vi "PWM Motor Control.vi"() -> ()   [LabVIEW 2010]
panel:
  out "Square":dynamicdata(graph)
  in  "Duty Cycle (%)":dbl=50.0
  in  "stop":bool
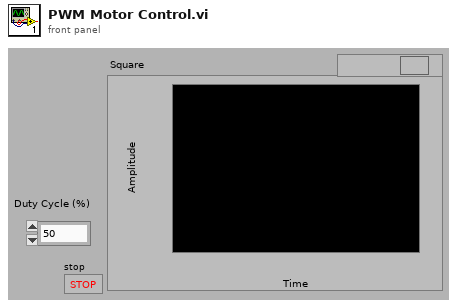
[diagram p1: front panel]
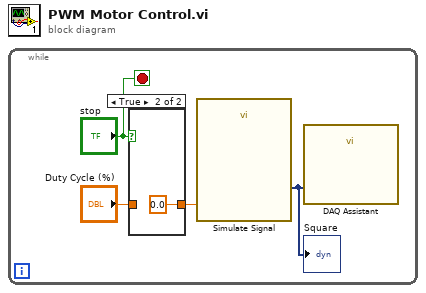
[diagram p0: block diagram]
diagram:
  n1 = while {
    stop <- "stop" stop-if-true
    n2 = case shown="True" "stop" {
      tunnel: "Duty Cycle (%)" -> [w5 _]
      tunnel: [w5 0.0 ("Duty Cycle (%)")] -> w1
      frame False {
      }
      frame True {
      }
    }
    n3 = call "Simulate Signal"("Duty Cycle (%)"=w1) -> ("Square"=w4:dynamicdata)  [unwired: 13 in, 1 out]
    "Square" <- w4
    n4 = call "DAQ Assistant"("data"=w4) -> ()  [unwired: 16 in, 3 out]
  }
